vi "Format Purchased Items.vi"(8 "error in (no error)":errorcluster, 10 "idvisits":i32, 11 "Provisional Line Items Corrected":T1[](array[typedef]) {"PriceIncDiscount (£)" format="%.2g"; "Discount(£)" format="%.2g"}) -> (0 "error out":errorcluster, 3 "Purchased Items Out":T2[](array[typedef]) {"TotalPriceIncludingDiscount" format="£%.2g"; "NumberOfUnits" format="%#.3g"; "TotalDiscount" format="£%.2g"})   [LabVIEW 2018, in "Main.lvlib"]
uses:
  Main.lvlib
  database/Purchased_Items--cluster.ctl
  receipt parsing/ReceiptItemInfo.ctl
  database/Database.lvlib
  receipt parsing/Receipt Parsing.lvlib
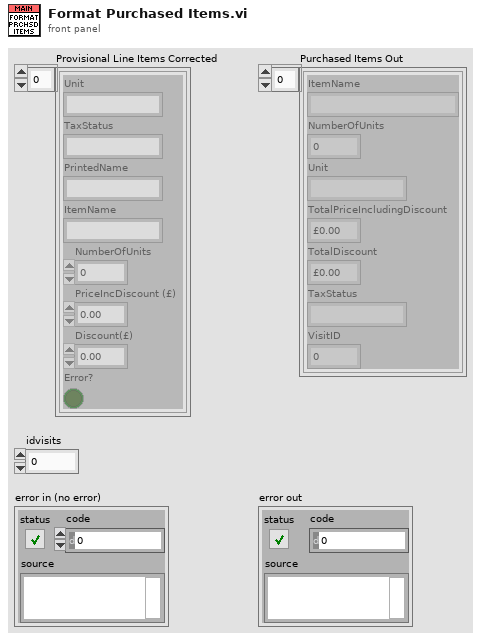
[diagram p1: front panel]
types:
  T1 = typedef "Receipt Parsing.lvlib/ReceiptItemInfo.ctl" = cluster{"Unit":string, "TaxStatus":string, "PrintedName":string, "ItemName":string, "NumberOfUnits":dbl, "PriceIncDiscount (£)":dbl, "Discount(£)":dbl, "Error?":bool}
  T2 = typedef "Database.lvlib/Purchased_Items--cluster.ctl" = cluster{"ItemName":string, "NumberOfUnits":dbl, "Unit":string, "TotalPriceIncludingDiscount":dbl, "TotalDiscount":dbl, "TaxStatus":string, "VisitID":i32}
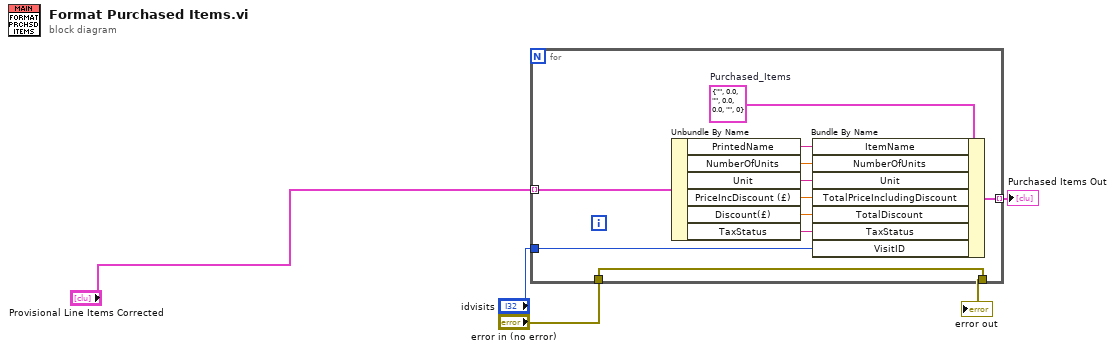
[diagram p0: block diagram]
diagram:
  n1 = for {
    tunnel: "Provisional Line Items Corrected" -> [w16] mode=indexing
    tunnel: [w14] -> w3 mode=indexing
    tunnel: "idvisits" -> [w7]
    tunnel: [w6] -> w5
    tunnel: "error in (no error)" -> [w6]
    w15 = T2 {"ItemName"="", "NumberOfUnits"=0.0, "Unit"="", "TotalPriceIncludingDiscount"=0.0, "TotalDiscount"=0.0, "TaxStatus"="", "VisitID"=0}  # Purchased_Items
    n2 = Unbundle By Name(w16) -> ("PrintedName"=w13:string, "NumberOfUnits"=w12:dbl, "Unit"=w11:string, "PriceIncDiscount (£)"=w10:dbl, "Discount(£)"=w9:dbl, "TaxStatus"=w8:string)
    n3 = Bundle By Name(cluster=w15, "ItemName"=w13, "NumberOfUnits"=w12, "Unit"=w11, "TotalPriceIncludingDiscount"=w10, "TotalDiscount"=w9, "TaxStatus"=w8, "VisitID"=w7) -> (w14:T2)
  }
  "error out" <- w5
  "Purchased Items Out" <- w3
